vi "Teleop.vi"(10 "Match Info":T1={"Autonomous Elapsed Seconds"=0.0, "TeleOp Elapsed Seconds"=0.0, "Disabled Elapsed Seconds"=0.0, "Visited Autonomous"=FALSE, "Visited TeleOp"=FALSE, "Visited Disabled"=FALSE, "Autonomous Settings"={"Autonomous Style"=enum."Independent", "VI Refnum"=refnum}}, 11 "Call Context":T2) -> ()   [LabVIEW 2014]
doc: "This VI is called for each TeleOp packet received from the DS where the robot is not disabled. It is often used to read from the joysticks and update I/O or to update setpoints for timed control loops. It should complete and return within 20 milliseconds or it may miss DS packets."
uses:
  <vilib>/Rock Robotics/WPI/DriverStation/WPI_DriverStationDerivedRobotMode.ctl
  <vilib>/Rock Robotics/WPI/DriverStation/WPI_DriverStationMatch Info.ctl
  <vilib>/Rock Robotics/WPI/RobotDrive/WPI_RobotDriveGetSetRefNum.vi
  <vilib>/Rock Robotics/WPI/Joystick/WPI_JoystickGetSetRefNum.vi
  Robot Global Data.vi
  <vilib>/Rock Robotics/Network Tables/SD Write Boolean Array.vi
  <vilib>/Rock Robotics/Network Tables/SD Write Numeric Array.vi
  <vilib>/Rock Robotics/Network Tables/SD Read Number.vi
  <vilib>/Rock Robotics/Network Tables/SD Write Boolean.vi
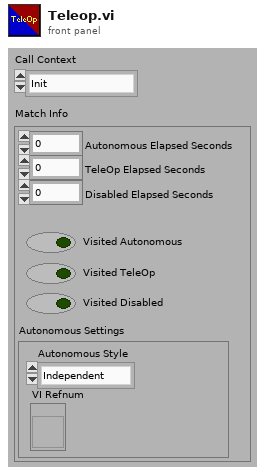
[diagram p1: front panel]
types:
  T1 = typedef "WPI_DriverStationMatch Info.ctl" = cluster{"Autonomous Elapsed Seconds":dbl, "TeleOp Elapsed Seconds":dbl, "Disabled Elapsed Seconds":dbl, "Visited Autonomous":bool, "Visited TeleOp":bool, "Visited Disabled":bool, "Autonomous Settings":cluster{"Autonomous Style":enum16{"Iterative", "Independent"}, "VI Refnum":refnum<vi>}}
  T2 = typedef "WPI_DriverStationDerivedRobotMode.ctl" = enum16{"Init", "Execute", "Stop"}
  T3 = typedef "WPI_JoystickDevRef.ctl" = cluster{"Device":T4}
  T4 = typedef "WPI_JoystickDeviceEnum.ctl" = enum16{"USB 0", "USB 1", "USB 2", "USB 3", "USB 4", "USB 5"}
  T5 = cluster{"POVs[0]":i16, "POVs[1]":i16, "POVs[2]":i16, "POVs[3]":i16, "POVs[4]":i16, "POVs[5]":i16, "POVs[6]":i16, "POVs[7]":i16, "POVs[8]":i16}
  T6 = cluster{"TopLeft":bool, "TopCenter":bool, "TopRight":bool, "MiddleRight":bool, "MiddleLeft":bool, "MiddleCenter":bool, "BottomRight":bool, "BottomLeft":bool, "BottomCenter":bool, "Top":bool, "Middle":bool, "Bottom":bool, "Left":bool, "Center":bool, "Right":bool}
  T7 = cluster{"Axes[0]":dbl, "Axes[1]":dbl, "Axes[2]":dbl, "Axes[3]":dbl, "Axes[4]":dbl, "Axes[5]":dbl, "Axes[6]":dbl, "Axes[7]":dbl, "Axes[8]":dbl}
  T8 = cluster{"Buttons[0]":bool, "Buttons[1]":bool, "Buttons[2]":bool, "Buttons[3]":bool, "Buttons[4]":bool, "Buttons[5]":bool, "Buttons[6]":bool, "Buttons[7]":bool, "Buttons[8]":bool}
  T9 = cluster{"Buttons[0]":bool, "Buttons[1]":bool, "Buttons[2]":bool, "Buttons[3]":bool, "Buttons[4]":bool, "Buttons[5]":bool, "Buttons[6]":bool, "Buttons[7]":bool, "Buttons[8]":bool, "Buttons[9]":bool, "Buttons[10]":bool, "Buttons[11]":bool, "Buttons[12]":bool, "Buttons[13]":bool, "Buttons[14]":bool, "Buttons[15]":bool}
  T10 = typedef "WPI_RobotDriveDevRef.ctl" = cluster{"DevStatus":errorcluster, "Motors[]":T11[], "Square Inputs":bool, "Max Output":dbl}
  T11 = typedef "WPI_MotorControlDeviceRef.ctl" = cluster{"DeviceStatus":errorcluster, "Type":T12, "PWM":cluster{"Controller":T13, "PWM Channel":T14, "DeadBand":T15}, "CAN":cluster{"Device Number":u8, "Control Mode":T16, "Semaphore":T17, "Max Vout":dbl, "TalonSRX Control Mode":T18}, "Invert":bool, "TransformRef":T19, "InvTransformRef":T19}
  T12 = typedef "WPI_MotorControlType.ctl" = enum16{"PWM", "CAN", "CANTalonSRX"}
  T13 = typedef "FPGA_TypedefDigitalModule.ctl" = enum16{"Controller 1"}
  T14 = typedef "FPGA_DIOPWMChannel.ctl" = enum8{"PWM 0", "PWM 1", "PWM 2", "PWM 3", "PWM 4", "PWM 5", "PWM 6", "PWM 7", "PWM 8", "PWM 9", "PWM MXP 0", "PWM MXP 1", "PWM MXP 2", "PWM MXP 3", "PWM MXP 4", "PWM MXP 5", "PWM MXP 6", "PWM MXP 7", "PWM MXP 8", "PWM MXP 9", "Invalid"}
  T15 = typedef "WPI_PWMDeadband.ctl" = cluster{"Name":string, "maxPositivePwm":i32, "minPositivePwm":i32, "centerPwm":i32, "maxNegativePwm":i32, "minNegativePwm":i32, "angularRange":u16}
  T16 = typedef "WPI_CANJaguar_ControlMode.ctl" = enum8{"Percent VBus", "Current", "Speed", "Position", "Voltage"}
  T17 = typedef "Semaphore RefNum" = refnum<k1>
  T18 = typedef "WPI_CANTalonSRX_APIControlMode.ctl" = enum8{"Percent VBus", "Speed", "Position", "Slave", "Unchanged / Invalid"}
  T19 = typedef "WPI_PWMTransform_ConPane.ctl" = refnum<vi>
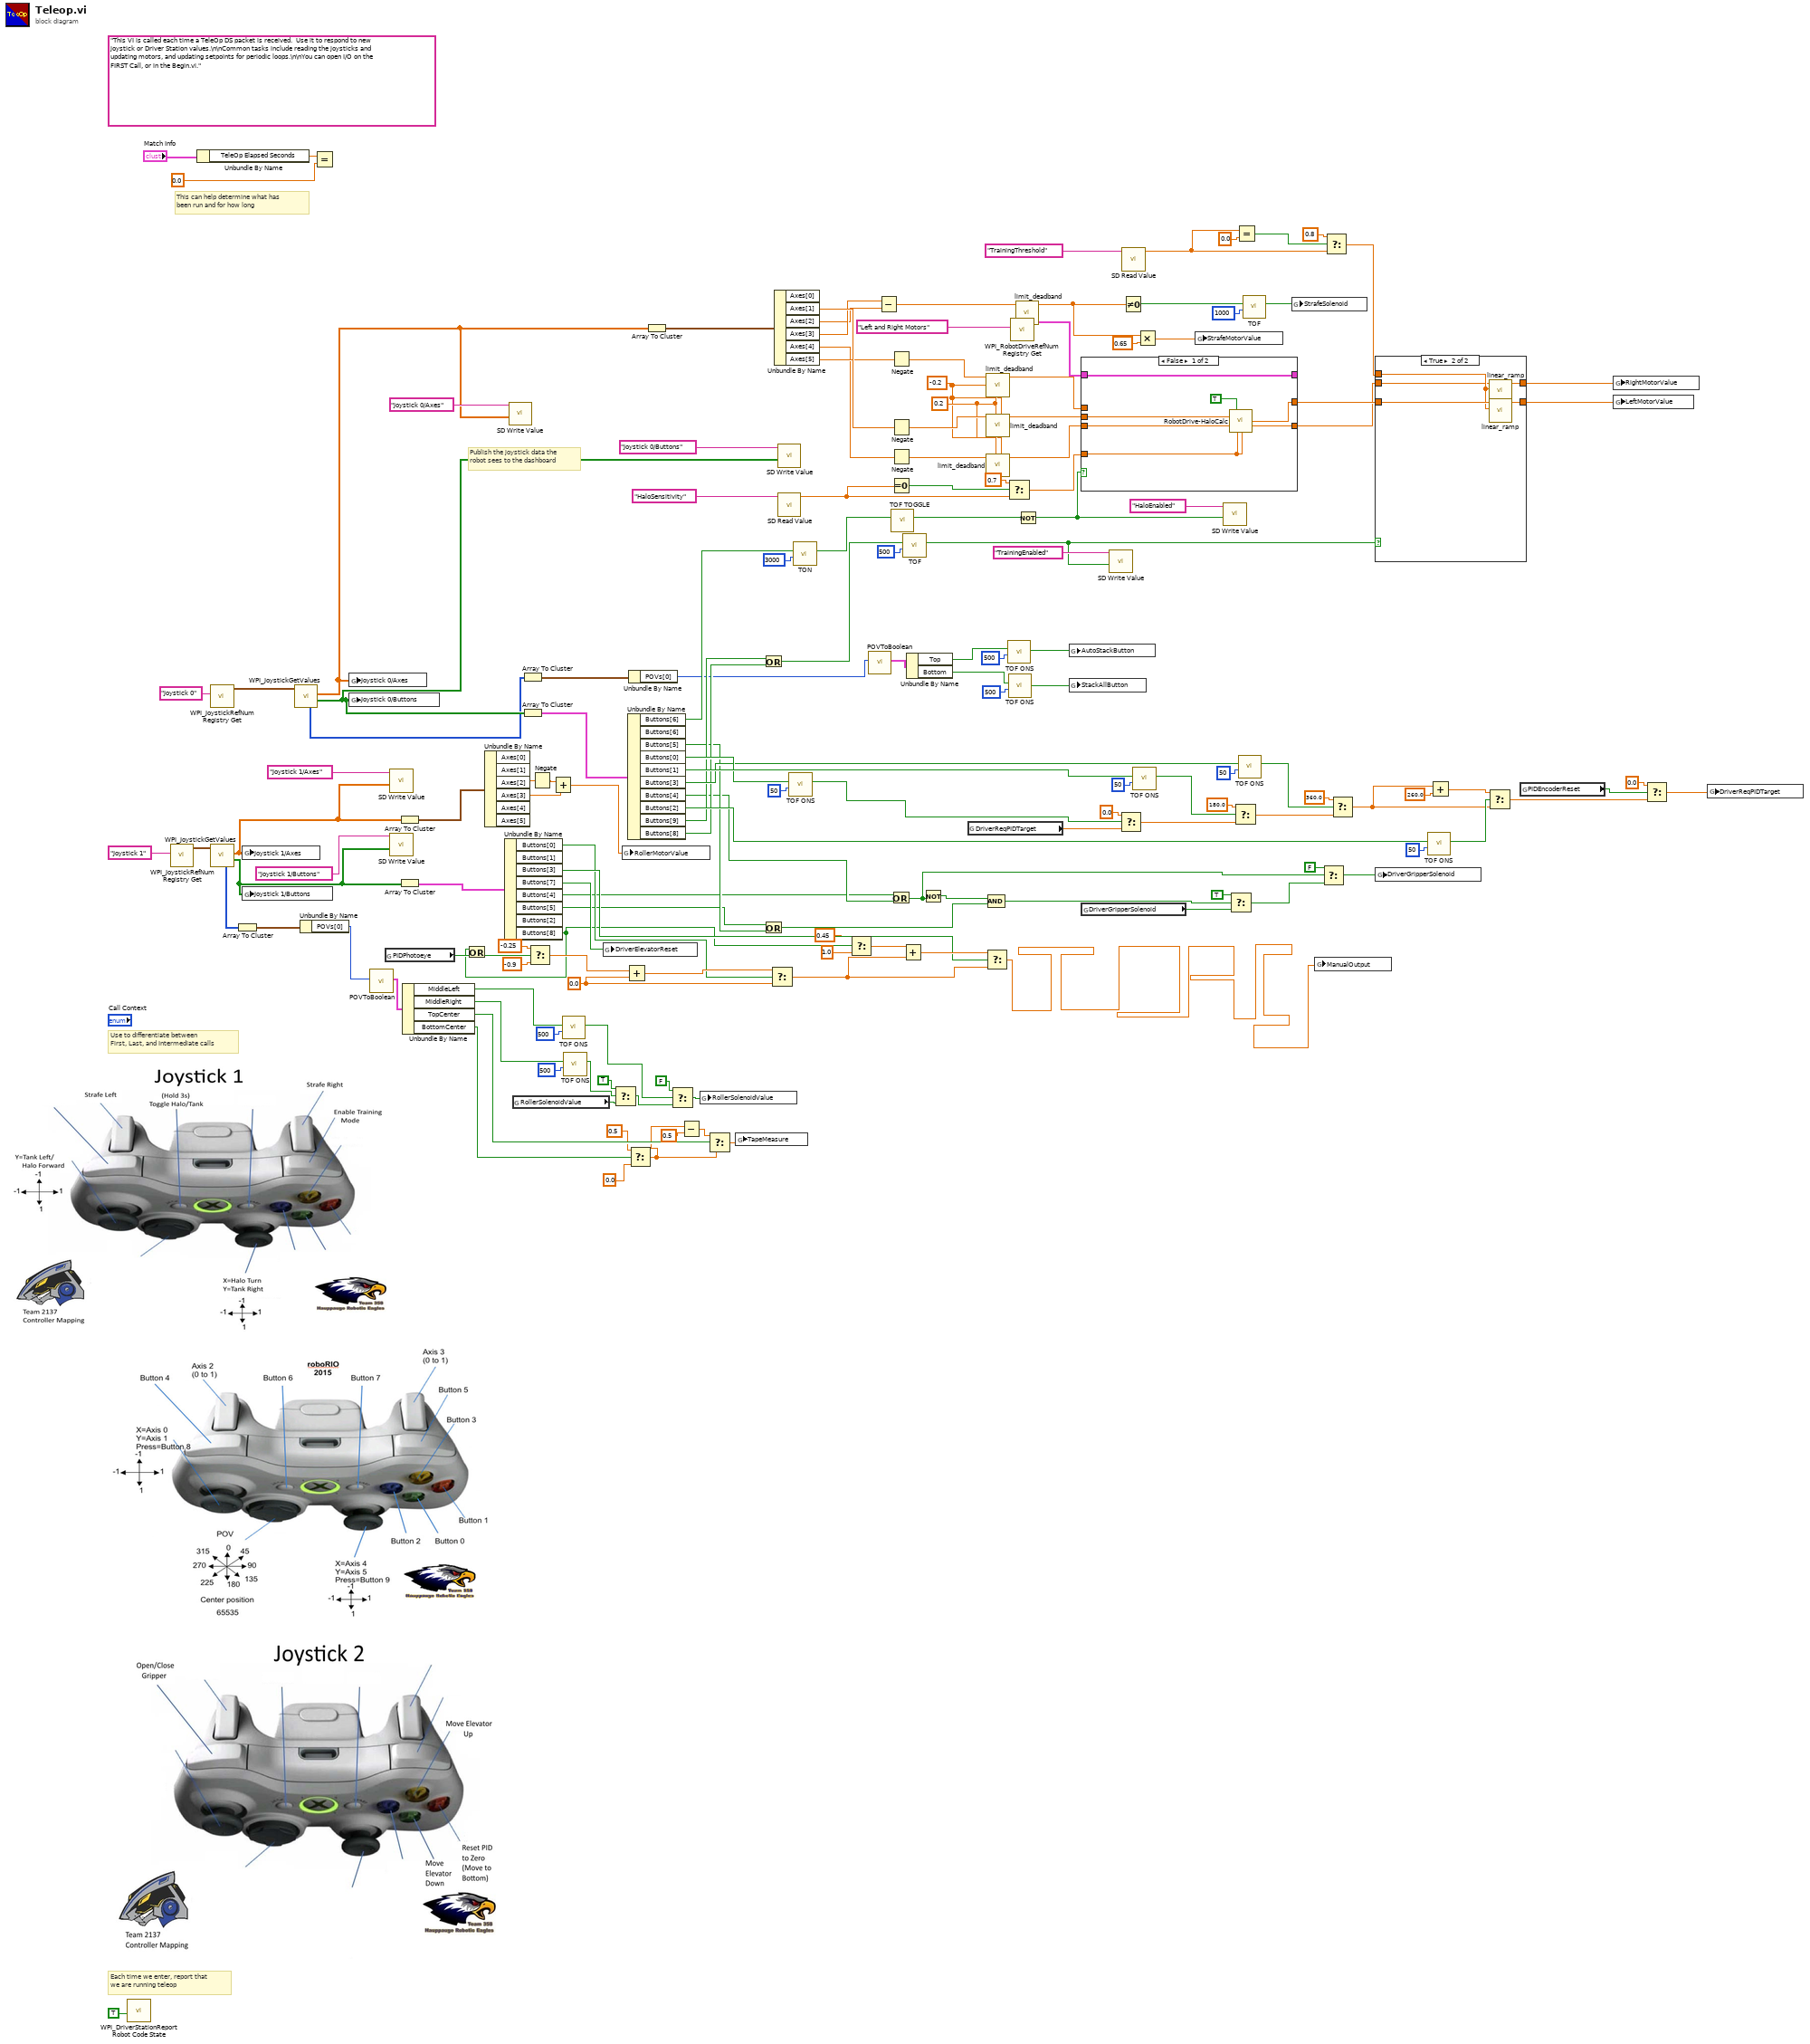
[diagram p0: block diagram]
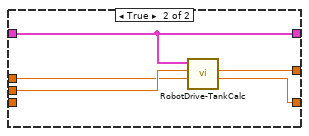
[diagram p3: hidden frame]
diagram:
  w59 = -0.2
  w60 = 0.2
  w125 = 0.0
  (unwired) "This VI is called each time a TeleOp DS packet is received.  Use it to respond to new joystick or Driver Station values.\n\nCommon tasks include reading the joysticks and updating motors, and updating setpoints for periodic loops.\n\nYou can open I/O on the FIRST Call, or in the Begin.vi."
  # "Publish the joystick data the\nrobot sees to the dashboard"
  # "Each time we enter, report that\nwe are running teleop"
  # "Use to differentiate between\nFirst, Last, and Intermediate calls"
  # "This can help determine what has\nbeen run and for how long"
  n1 = call <vilib>:"WPI_DriverStationReport Robot Code State.vi"("TeleOp"=TRUE ("Autonomous")) -> ()  [unwired: 10 in, 1 out]
  n2 = call <vilib>:"WPI_JoystickRefNum Registry Get.vi"("refnum name"="Joystick 1") -> ("JoystickDevRef"=w136:T3)  [unwired: 1 in, 9 out]
  n3 = Unbundle By Name("Match Info") -> ("TeleOp Elapsed Seconds"=w128:dbl)
  n4 = call <vilib>:"WPI_JoystickRefNum Registry Get.vi"("refnum name"="Joystick 0") -> ("JoystickDevRef"=w158:T3)  [unwired: 1 in, 9 out]
  n5 = call <vilib>:"WPI_JoystickGetValues.vi"("JoystickDevRef"=w136) -> ("Buttons"=w131:bool[], "Axes"=w132:dbl[], "POVs"=w35:i16[])  [unwired: 6 in, 2 out]
  n6 = Array To Cluster(array=w35) -> (cluster=w34:T5)
  n7 = global write "Robot Global Data.vi" "Joystick 1/Axes"(w132) -> ()
  n8 = global write "Robot Global Data.vi" "Joystick 1/Buttons"(w131) -> ()
  n9 = call <vilib>:"WPI_JoystickGetValues.vi"("JoystickDevRef"=w158) -> ("Buttons"=w129:bool[], "Axes"=w130:dbl[], "POVs"=w83:i16[])  [unwired: 6 in, 2 out]
  n10 = Unbundle By Name(w34) -> ("POVs[0]"=w33:i16)
  n11 = Equal?(x=w128, y=0.0) -> ()  [unwired: 1 out]
  n12 = global write "Robot Global Data.vi" "Joystick 0/Axes"(w130) -> ()
  n13 = global write "Robot Global Data.vi" "Joystick 0/Buttons"(w129) -> ()
  n14 = call "POVToBoolean.vi"("Input"=w33) -> ("Output"=w32:T6)  [unwired: 10 in]
  n15 = global read "Robot Global Data.vi" "PIDPhotoeye"() -> (w70:bool)
  n16 = call-poly <vilib>:"SD Write Value.vi"("Numeric Array"=w132, "Name"="Joystick 1/Axes") -> ()  [unwired: 8 in, 2 out]
  n17 = call-poly <vilib>:"SD Write Value.vi"("Boolean Array"=w131, "Name"="Joystick 1/Buttons") -> ()  [unwired: 8 in, 2 out]
  n18 = Array To Cluster(array=w132) -> (cluster=w133:T7)
  n19 = Array To Cluster(array=w131) -> (cluster=w126:T8)
  n20 = Unbundle By Name(w32) -> ("MiddleLeft"=w30:bool, "MiddleRight"=w31:bool, "TopCenter"=w18:bool, "BottomCenter"=w13:bool)
  n21 = Unbundle By Name(w133) -> ("Axes[2]"=w40:dbl, "Axes[3]"=w21:dbl)  [unwired: 4 out]
  n22 = Unbundle By Name(w126) -> ("Buttons[0]"=w112:bool, "Buttons[3]"=w113:bool, "Buttons[7]"=w91:bool, "Buttons[4]"=w45:bool, "Buttons[5]"=w53:bool, "Buttons[8]"=w3:bool)  [unwired: 2 out]
  n23 = Or(x=w3, y=w70) -> (x .or. y?=w20:bool)
  n24 = call-poly <vilib>:"SD Write Value.vi"("Numeric Array"=w130, "Name"="Joystick 0/Axes") -> ()  [unwired: 8 in, 2 out]
  n25 = global read "Robot Global Data.vi" "RollerSolenoidValue"() -> (w27:bool)
  n26 = Array To Cluster(array=w83) -> (cluster=w86:T5)
  n27 = Array To Cluster(array=w129) -> (cluster=w58:T9)
  n28 = Select(t=-0.25, s=w20, f=-0.9 ("x")) -> (s? t:f=w67:dbl)
  n29 = Negate(x=w40) -> (-x=w22:dbl)
  n30 = Add(x=w22, y=w21) -> (x+y=w39:dbl)
  n31 = call "TOF ONS.vi"("Delay (ms)"=u32 500, "Input"=w30) -> ("Output"=w23:bool)  [unwired: 9 in]
  n32 = call "TOF ONS.vi"("Delay (ms)"=u32 500, "Input"=w31) -> ("Output"=w25:bool)  [unwired: 9 in]
  n33 = global write "Robot Global Data.vi" "DriverElevatorReset"(w91) -> ()
  n34 = Select(t=TRUE, s=w25, f=w27) -> (s? t:f=w28:bool)
  n35 = global write "Robot Global Data.vi" "RollerMotorValue"(w39) -> ()
  n36 = Add(x=w67, y=w125) -> (x+y=w124:dbl)
  n37 = Unbundle By Name(w58) -> ("Buttons[6]"=w142:bool, "Buttons[5]"=w54:bool, "Buttons[0]"=w106:bool, "Buttons[1]"=w109:bool, "Buttons[3]"=w102:bool, "Buttons[4]"=w52:bool, "Buttons[2]"=w92:bool, "Buttons[9]"=w57:bool, "Buttons[8]"=w56:bool)  [unwired: 1 out]
  n38 = Unbundle By Name(w86) -> ("POVs[0]"=w12:i16)
  n39 = Select(t=0.5 ("y"), s=w13, f=0.0) -> (s? t:f=w8:dbl)
  n40 = Array To Cluster(array=w130) -> (cluster=w154:T7)
  n41 = Select(t=FALSE, s=w23, f=w28) -> (s? t:f=w29:bool)
  n42 = Subtract(x=w8, y=0.5) -> (x-y=w17:dbl)
  n43 = global write "Robot Global Data.vi" "RollerSolenoidValue"(w29) -> ()
  n44 = Select(t=w17, s=w18, f=w8) -> (s? t:f=w19:dbl)
  n45 = global write "Robot Global Data.vi" "TapeMeasure"(w19) -> ()
  n46 = Or(x=w57, y=w56) -> (x .or. y?=w55:bool)
  n47 = Or(x=w53, y=w54) -> (x .or. y?=w44:bool)
  n48 = Select(t=w124, s=w112, f=w125) -> (s? t:f=w42:dbl)
  n49 = Unbundle By Name(w154) -> ("Axes[1]"=w153:dbl, "Axes[2]"=w147:dbl, "Axes[3]"=w148:dbl, "Axes[4]"=w139:dbl, "Axes[5]"=w151:dbl)  [unwired: 1 out]
  n50 = call-poly <vilib>:"SD Write Value.vi"("Boolean Array"=w129, "Name"="Joystick 0/Buttons") -> ()  [unwired: 8 in, 2 out]
  n51 = call-poly <vilib>:"SD Read Value.vi"("Name"="HaloSensitivity") -> ("Numeric"=w80:dbl)  [unwired: 8 in, 2 out]
  n52 = call "TOF ONS.vi"("Delay (ms)"=u32 50, "Input"=w106) -> ("Output"=w38:bool)  [unwired: 9 in]
  n53 = call "TON.vi"("Delay (ms)"=u32 3000, "Input"=w142) -> ("Output"=w143:bool)  [unwired: 9 in]
  n54 = Select(t=0.45, s=w3, f=1.0 ("x")) -> (s? t:f=w2:dbl)
  n55 = call "POVToBoolean.vi"("Input"=w12) -> ("Output"=w11:T6)  [unwired: 10 in]
  n56 = Subtract(x=w148, y=w147) -> (x-y=w149:dbl)
  n57 = Negate(x=w151) -> (-x=w150:dbl)
  n58 = Negate(x=w153) -> (-x=w152:dbl)
  n59 = Negate(x=w139) -> (-x=w140:dbl)
  n60 = Equal To 0?(x=w80) -> (x = 0?=w82:bool)
  n61 = Or(x=w45, y=w52) -> (x .or. y?=w1:bool)
  n62 = call "TOF TOGGLE.vi"("Input"=w143) -> ("Output"=w114:bool)  [unwired: 10 in]
  n63 = Add(x=w2, y=w42) -> (x+y=w123:dbl)
  n64 = call "TOF.vi"("Delay (ms)"=u32 500, "Input"=w55) -> ("Output"=w72:bool)  [unwired: 9 in]
  n65 = Unbundle By Name(w11) -> ("Top"=w10:bool, "Bottom"=w9:bool)
  n66 = Not(x=w1) -> (.not. x?=w43:bool)
  n67 = global read "Robot Global Data.vi" "DriverReqPIDTarget"() -> (w71:dbl)
  n68 = Select(t=w123, s=w113, f=w42) -> (s? t:f=w41:dbl)
  n69 = call "limit_deadband.vi"("lower limit"=w59, "upper limit"=w60, "Val"=w150) -> ("Val Out"=w144:dbl)  [unwired: 8 in]
  n70 = call "limit_deadband.vi"("lower limit"=w59, "upper limit"=w60, "Val"=w152) -> ("Val Out"=w145:dbl)  [unwired: 8 in]
  n71 = call "limit_deadband.vi"("lower limit"=w59, "upper limit"=w60, "Val"=w140) -> ("Val Out"=w138:dbl)  [unwired: 8 in]
  n72 = Compound Arithmetic op=AND(w43, w44) -> (w51:bool)
  n73 = Select(t=0.7, s=w82, f=w80) -> (s? t:f=w79:dbl)
  n74 = call "TOF ONS.vi"("Delay (ms)"=u32 500, "Input"=w10) -> ("Output"=w6:bool)  [unwired: 9 in]
  n75 = call "TOF ONS.vi"("Delay (ms)"=u32 500, "Input"=w9) -> ("Output"=w7:bool)  [unwired: 9 in]
  n76 = call <vilib>:"WPI_RobotDriveRefNum Registry Get.vi"("refnum name"="Left and Right Motors") -> ("RobotDriveDevRef"=w146:T10)  [unwired: 1 in, 9 out]
  n77 = call "limit_deadband.vi"("Val"=w149) -> ("Val Out"=w61:dbl)  [unwired: 10 in]
  n78 = Not(x=w114) -> (.not. x?=w98:bool)
  n79 = global write "Robot Global Data.vi" "AutoStackButton"(w6) -> ()
  n80 = global write "Robot Global Data.vi" "StackAllButton"(w7) -> ()
  n81 = case shown="False" w98 {
    tunnel: w146 -> [w165 w169]
    tunnel: [w168 w173] -> w120
    tunnel: [w167 w172] -> w117
    tunnel: w145 -> [w166 w171]
    tunnel: w144 -> [_ w170]
    tunnel: w79 -> [w162 _]
    tunnel: [w165 w169] -> _
    tunnel: w138 -> [w163 _]
    frame False {
      n82 = call "RobotDrive-HaloCalc.vi"("QwikTurnButton"=TRUE, "Left axis value"=w166, "Right axis value"=w163, "Sensitivity"=w162, "QuikTurn Sensitivity"=w162) -> ("Left Output"=w168:dbl, "Right Output"=w167:dbl)  [unwired: 9 in]
    }
    frame True {
      n83 = call "RobotDrive-TankCalc.vi"("Right axis value"=w170, "Left axis value"=w171, "RobotDriveDevRef"=w169) -> ("Right motor value"=w172:dbl, "Left motor value"=w173:dbl)  [unwired: 7 in]
    }
  }
  n84 = global read "Robot Global Data.vi" "DriverGripperSolenoid"() -> (w50:bool)
  n85 = call-poly <vilib>:"SD Write Value.vi"("Boolean"=w72, "Name"="TrainingEnabled") -> ()  [unwired: 8 in, 2 out]
  n86 = Select(t=0.0, s=w38, f=w71) -> (s? t:f=w110:dbl)
  n87 = call-poly <vilib>:"SD Read Value.vi"("Name"="TrainingThreshold") -> ("Numeric"=w75:dbl)  [unwired: 8 in, 2 out]
  n88 = Not Equal To 0?(x=w61) -> (x != 0?=w64:bool)
  n89 = call "TOF ONS.vi"("Delay (ms)"=u32 50, "Input"=w109) -> ("Output"=w107:bool)  [unwired: 9 in]
  n90 = Multiply(x=w61, y=0.65) -> (x*y=w66:dbl)
  n91 = global write "Robot Global Data.vi" "StrafeMotorValue"(w66) -> ()
  n92 = call-poly <vilib>:"SD Write Value.vi"("Boolean"=w98, "Name"="HaloEnabled") -> ()  [unwired: 8 in, 2 out]
  n93 = Select(t=TRUE, s=w51, f=w50) -> (s? t:f=w48:bool)
  n94 = Select(t=180.0, s=w107, f=w110) -> (s? t:f=w101:dbl)
  n95 = Equal?(x=w75, y=0.0) -> (x = y?=w77:bool)
  n96 = call "TOF ONS.vi"("Delay (ms)"=u32 50, "Input"=w102) -> ("Output"=w99:bool)  [unwired: 9 in]
  n97 = call "TOF.vi"("Delay (ms)"=u32 1000, "Input"=w64) -> ("Output"=w62:bool)  [unwired: 9 in]
  n98 = global write "Robot Global Data.vi" "StrafeSolenoid"(w62) -> ()
  n99 = global write "Robot Global Data.vi" "ManualOutput"(w41) -> ()
  n100 = Select(t=FALSE, s=w1, f=w48) -> (s? t:f=w46:bool)
  n101 = Select(t=0.8, s=w77, f=w75) -> (s? t:f=w74:dbl)
  n102 = Select(t=360.0, s=w99, f=w101) -> (s? t:f=w94:dbl)
  n103 = case shown="True" w72 {
    tunnel: [w175 w179] -> w119
    tunnel: w120 -> [w175 w180]
    tunnel: [w174 w176] -> w118
    tunnel: w117 -> [w174 w177]
    tunnel: w74 -> [_ w178]
    frame False {
    }
    frame True {
      n104 = call "linear_ramp.vi"("filter const (dx/dt)"=w178, "input"=w177) -> ("output"=w176:dbl)  [unwired: 9 in]
      n105 = call "linear_ramp.vi"("filter const (dx/dt)"=w178, "input"=w180) -> ("output"=w179:dbl)  [unwired: 9 in]
    }
  }
  n106 = global write "Robot Global Data.vi" "DriverGripperSolenoid"(w46) -> ()
  n107 = call "TOF ONS.vi"("Delay (ms)"=u32 50, "Input"=w92) -> ("Output"=w96:bool)  [unwired: 9 in]
  n108 = Add(x=w94, y=260.0) -> (x+y=w95:dbl)
  n109 = Select(t=w95, s=w96, f=w94) -> (s? t:f=w90:dbl)
  n110 = global read "Robot Global Data.vi" "PIDEncoderReset"() -> (w88:bool)
  n111 = global write "Robot Global Data.vi" "RightMotorValue"(w118) -> ()
  n112 = global write "Robot Global Data.vi" "LeftMotorValue"(w119) -> ()
  n113 = Select(t=0.0, s=w88, f=w90) -> (s? t:f=w89:dbl)
  n114 = global write "Robot Global Data.vi" "DriverReqPIDTarget"(w89) -> ()
